vi "QuadratureEncoder.vi"() -> ()   [LabVIEW 2016]
doc: "DESCRIPTION:\nThis VI measures the rotation of a quadrature encoder. The quadrature encoder produces 96 pulses/revolution. \n\nNOTE: This VI only works with the BNC-2120 Connector Assembly.\n\n\n\nINSTRUCTIONS:\nEnter the appropriate device and counter number. Wire the BNC-2120 appropriately for the specified counter. By rotating the BNC quadrature encoder knob the vi will display the number of pulses and degrees rotated.\n\n\nKEY PARAMETERS:\n* device (Counter Group Config.vi): the device number you assigned to the E-Series DAQ device during configuration.\n* counter: (Counter Group Config.vi) the counter on the E-Series DAQ device you wish to use, either 0 or 1.\n\n\nI/O CONNECTIONS OVERVIEW:\nOn the BNC-2120, connect the CLK signal to the Source of the counter being used. \n For CTR0, connect CLK to CTR Source 0 (PFI8).\n For CTR1, connect CLK to CTR Source 1 (PFI3).\n\nConnect UP/DN signal to the direction line of the DAQ-STC as follows:\n For CTR0, connect UP/DN to DIO6.\n For CTR1, connect UP/DN to DIO7."
uses:
  <vilib>/myRIO/Common/Instrument Driver Framework/myRIO v1.0/Encoder/typedefs/Encoder Signal Mode.ctl
  <vilib>/myRIO/Instrument Drivers/Onboard IO/Encoder/typedefs/Encoder Reference.ctl
  <vilib>/myRIO/Common/Instrument Driver Framework/Utilities/typedefs/myRIO Generic Hardware Reference.ctl
  <vilib>/myRIO/Common/Instrument Driver Framework/Utilities/typedefs/Hardware Version Enum.ctl
  <vilib>/myRIO/Common/Instrument Driver Framework/Utilities/typedefs/myRIO v1.0 Reference.ctl
  <vilib>/myRIO/Common/Instrument Driver Framework/Utilities/typedefs/Generic FPGA Reference.ctl
  <vilib>/myRIO/Common/Instrument Driver Framework/myRIO v1.0/Encoder/typedefs/Encoder Channels Enum.ctl
  <vilib>/myRIO/Common/Instrument Driver Framework/myRIO v1.0/Encoder/typedefs/Encoder Configuration v1.0.ctl
  <vilib>/userdefined/High Color/nirio_resource_hc.ctl
  <vilib>/myRIO/Common/Instrument Driver Framework/Utilities/vis/Is FPGA Ref Available.vi
  <vilib>/myRIO/Common/Instrument Driver Framework/myRIO v1.0/Encoder/vis/myRIO v1.1 Open Encoder.vi
  <vilib>/myRIO/Instrument Drivers/Onboard IO/Encoder/vis/Read.vi
  <vilib>/myRIO/Common/Instrument Driver Framework/Utilities/vis/Validate Channels.vi
  <vilib>/myRIO/Common/Instrument Driver Framework/myRIO v1.0/Encoder/vis/myRIO v1.0 Reserve Encoder.vi
  <vilib>/myRIO/Common/Instrument Driver Framework/myRIO v1.0/UART/vis/myRIO v1.0 Close UART.vi
  <vilib>/myRIO/Common/Instrument Driver Framework/myRIO v1.0/Encoder/vis/myRIO v1.0 Build MUX Configuration Encoder.vi
  <vilib>/myRIO/Common/Instrument Driver Framework/myRIO v1.0/Resource Manager/vis/myRIO v1.0 Reserve Channel List.vi
  <vilib>/myRIO/Common/Instrument Driver Framework/myRIO v1.0/Resource Manager/vis/myRIO v1.0 Create Configuration List.vi
  <vilib>/myRIO/Common/Instrument Driver Framework/myRIO v1.0/Resource Manager/vis/myRIO v1.0 Reserve Channel.vi
  <vilib>/myRIO/Common/Instrument Driver Framework/myRIO v1.0/Resource Manager/vis/myRIO v1.0 Unreserve Channel.vi
  <vilib>/myRIO/Common/Instrument Driver Framework/myRIO v1.0/Resource Manager/vis/myRIO v1.0 Build Mutex Name.vi
  <vilib>/Utility/VariantDataType/GetNumericInfo.vi
  <vilib>/Utility/error.llb/Error Cluster From Error Code.vi
  <vilib>/myRIO/Common/Instrument Driver Framework/myRIO v1.0/myRIO v1.1 Open.vi
  <vilib>/myRIO/Common/Instrument Driver Framework/Utilities/vis/IO Manager.vi
  <vilib>/myRIO/Common/Instrument Driver Framework/Utilities/vis/Configuration Manager.vi
  <vilib>/myRIO/Common/Instrument Driver Framework/myRIO v1.0/Resource Manager/vis/myRIO v1.0 Configure IO.vi
  <vilib>/myRIO/Common/Instrument Driver Framework/myRIO v1.0/myRIO v1.0 Close.vi
  <vilib>/myRIO/Common/Instrument Driver Framework/myRIO v1.0/Encoder/vis/myRIO v1.0 Configure Encoder.vi
  <vilib>/myRIO/Common/Instrument Driver Framework/myRIO v1.0/Encoder/vis/myRIO v1.0 Read Encoder.vi
  <vilib>/myRIO/Common/Instrument Driver Framework/Utilities/vis/FPGA Ref Manager.vi
  <vilib>/myRIO/Common/Instrument Driver Framework/myRIO v1.0/myRIO v1.0 Reset FPGA.vi
  <vilib>/myRIO/Common/Instrument Driver Framework/myRIO v1.0/IRQ/vis/myRIO v1.0 IRQ Info FGV.vi
  <vilib>/myRIO/Common/Instrument Driver Framework/myRIO v1.0/IRQ/vis/myRIO v1.0 Timer IRQ Info FGV.vi
  <vilib>/myRIO/Common/Instrument Driver Framework/myRIO v1.0/IRQ/vis/myRIO v1.0 ISR Agent.vi
  <vilib>/myRIO/Express VI/Onboard IO/Encoder/Encoder Express VI.xnode
  <vilib>/myRIO/Instrument Drivers/Onboard IO/Encoder/vis/myRIO Encoder Open.xnode
  <vilib>/myRIO/Common/Instrument Driver Framework/myRIO v1.0/Encoder/typedefs/Encoder Count Direction Enum.ctl
  <vilib>/myRIO/Instrument Drivers/Utilities/Utilities.lvlib
  <vilib>/myRIO/Instrument Drivers/Onboard IO/Encoder/Encoder.lvlib
panel:
  out "Distance Travelled":dbl
  out "Degrees":dbl(knob) scale=0.0..360.0 scale format="%#.1f"
  out "Number of Revolutions":dbl
  out "Total Degrees Rotated":dbl format="%.2f"
  out "CLK pulses":i32 caption="CLK pulses 2"
  in  "stop":bool
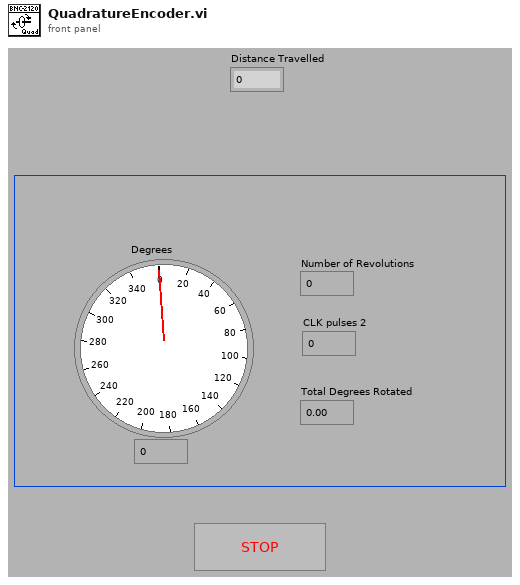
[diagram p1: front panel]
types:
  T1 = typedef "Encoder.lvlib/Encoder Reference.ctl" = cluster{"myRIO Reference":T2, "Encoder Channels Enum":T6}
  T2 = typedef "myRIO Generic Hardware Reference.ctl" = cluster{"myRIO Model":T3, "myRIO Hardware Reference":T4}
  T3 = typedef "Hardware Version Enum.ctl" = enum16{"Unknown", "myRIO-1900", "myRIO-1950", "roboRIO", "NI ELVIS RIO CM"}
  T4 = typedef "myRIO v1.0 Reference.ctl" = cluster{"Generic FPGA Reference":T5, "Allow multiple opens":bool}
  T5 = typedef "Generic FPGA Reference.ctl" = refnum<k20>
  T6 = typedef "Encoder Channels Enum.ctl" = enum16{"Not Connected", "C/ENC0", "C/ENC1", "A/ENC", "B/ENC", "DIO/ENC0", "DIO/ENC1", "DIO/ENC2", "DIO/ENC3", "DIO/ENC4"}
  T7 = typedef "Encoder Signal Mode.ctl" = enum16{"Quadrature phase signal", "Step and direction signal"}
  T8 = typedef "nirio_resource_hc.ctl" = tag
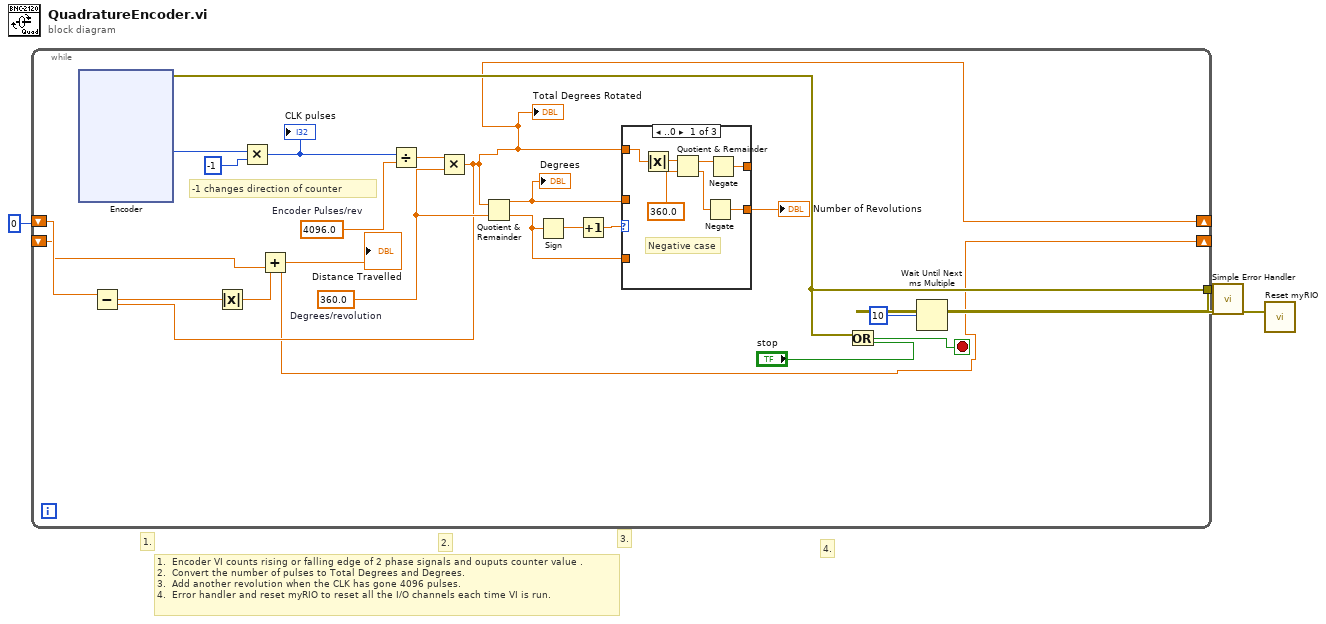
[diagram p0: block diagram]
diagram:
  # "4."
  # "3."
  # "2."
  # "1."
  # "1.  Encoder VI counts rising or falling edge of 2 phase signals and ouputs counter value .\n2.  Convert the number of pulses to Total Degrees and Degrees.\n3.  Add another revolution when the CLK has gone 4096 pulses.\n4.  Error handler and reset myRIO to reset all the I/O channels each time VI is run."
  n1 = while {
    tunnel: [w18] -> w2
    shift-right: [w10] -> _
    shift-left: 0 -> [w11]
    shift-right: [w4] -> _
    shift-left: _ -> [w7]
    stop <- w5 stop-if-true
    w15 = 4096.0  # Encoder Pulses/rev
    w12 = 360.0  # Degrees/revolution
    # "-1 changes direction of counter"
    n2 = xnode "Encoder"() -> ("Counter Value"=w16:i32, "error out"=w18:errorcluster)  [unwired: 2 in, 2 out]
    n3 = Multiply(x=w16, y=-1) -> (x*y=w14:i32)
    "CLK pulses" <- w14
    n4 = Divide(x=w14, y=w15) -> (x/y=w13:dbl)
    n5 = Multiply(x=w13, y=w12) -> (x*y=w10:dbl)
    "Total Degrees Rotated" <- w10
    n6 = Subtract(x=w11, y=w10) -> (x-y=w9:dbl)
    n7 = Absolute Value(x=w9) -> (abs(x)=w8:dbl)
    n8 = Add(x=w8, y=w7) -> (x+y=w4:dbl)
    "Distance Travelled" <- w4
    n9 = Quotient & Remainder(x=w10, y=w12) -> (x-y*floor(x/y)=w19:dbl, floor(x/y)=w20:dbl)
    "Degrees" <- w19
    n10 = Sign(1:w20) -> (0:w23:dbl)
    n11 = Increment(x=w23) -> (x+1=w22:dbl)
    n12 = case shown="..0" w22 {
      tunnel: w10 -> [w77 _ _]
      tunnel: w19 -> [_ w79 w81]
      tunnel: [w72 w78 w80] -> w21
      tunnel: [w71 w79 w81] -> _
      tunnel: w20 -> [_ w78 w80]
      frame ..0 {
        # "Negative case"
        n13 = Absolute Value(x=w77) -> (abs(x)=w76:dbl)
        n14 = Quotient & Remainder(x=w76, y=360.0) -> (x-y*floor(x/y)=w75:dbl, floor(x/y)=w73:dbl)
        n15 = Negate(x=w73) -> (-x=w72:dbl)
        n16 = Negate(x=w75) -> (-x=w71:dbl)
      }
      frame 1 {
      }
      frame 2.. {
      }
    }
    "Number of Revolutions" <- w21
    n17 = Or(x=w18, y="stop") -> (x .or. y?=w5:bool)
    n18 = Wait Until Next ms Multiple(millisecond multiple=10) -> ()  [unwired: 1 out]
  }
  n19 = call <vilib>:"Simple Error Handler.vi"("error in (no error)"=w2) -> ("error out"=w3:errorcluster)  [unwired: 4 in, 4 out]
  n20 = call <vilib>:"Reset myRIO.vi"("error in (no error)"=w3) -> ()  [unwired: 10 in, 1 out]
